vi "Read.vi"(8 "error in (no error)":errorcluster, 11 "Saving OO in":refnum<class "Saving OO.lvclass">) -> (0 "error out":errorcluster, 2 "Data":string[][](array[string]), 3 "Saving OO out":refnum<class "Saving OO.lvclass">)   [LabVIEW 2020, in "Saving OO.lvclass"]
uses:
  Saving OO.lvclass
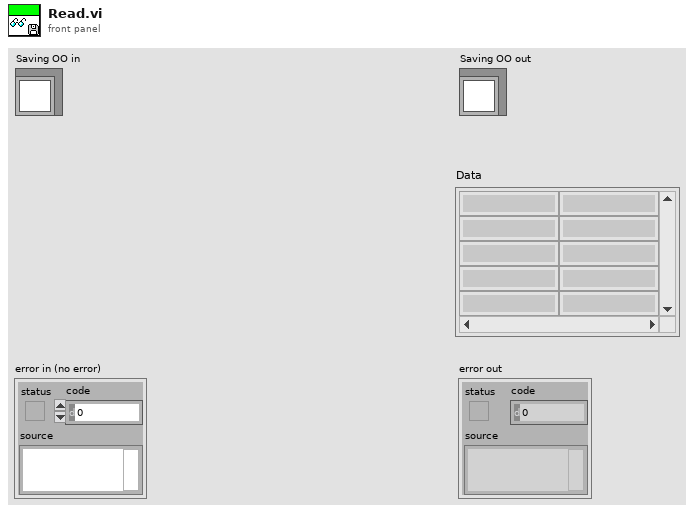
[diagram p1: front panel]
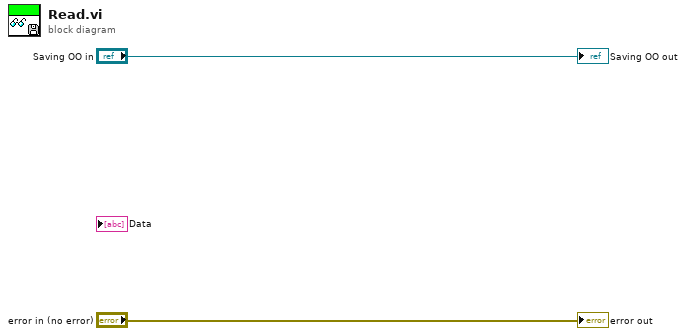
[diagram p0: block diagram]
diagram:
  "error out" <- "error in (no error)"
  "Saving OO out" <- "Saving OO in"
